vi "MicroblazeHostExample.vi"() -> ()   [LabVIEW 2015]
uses:
  <vilib>/userdefined/High Color/nirio_resource_hc.ctl
  <vilib>/FPGAPlugInAG/PXIe-6592R/niLvFpga_Open_PXIe-6592R.vi
  <vilib>/rvi/interface/common/dynamic/niFpgaDynamicAddResources.vi
  <vilib>/FPGAPlugInAG/Dynamic/niLvFpga_Reset_Dynamic.vi
  <vilib>/FPGAPlugInAG/Dynamic/niLvFpga_Download_Dynamic.vi
  <vilib>/FPGAPlugInAG/Dynamic/niLvFpga_Run_Dynamic.vi
  <vilib>/Utility/error.llb/Error Cluster From Error Code.vi
  <vilib>/rvi/errors/niLvFpgaAdjustHostInterfaceError.vi
  <vilib>/FPGAPlugInAG/Dynamic/niLvFpga_Close_Dynamic.vi
  <vilib>/rvi/interface/nirviOpenFPGA/nirviOpenFPGA.xnode
  FPGA Bitfiles/working/Microblaze.lvbitx
  <vilib>/rvi/interface/nirviMethod/nirviMethod.xnode
  <vilib>/rvi/interface/nirviReadWriteControl/nirviReadWriteControl.xnode
  <vilib>/rvi/interface/nirviCloseFPGA/nirviCloseFPGA.xnode
  <vilib>/rvi/interface/Simulation/niFpgaSimulationCallBeginRW.vi
  NiFpgaLv.dll
panel:
  in  "Flush Console":bool
  out "error out":errorcluster
  in  "FPGA Resource Name":T1="PXI1Slot6"
  out "UART Console":string="Goodbye cruel World\r\n"
  out "C":u32=12
  in  "B":u32=6
  in  "A":u32=2
  in  "C Code Executable to Download":path=path "C:/Users/8135cont24/Documents/CodeDistribution/LVFPGAHost/MicroBlazeELFFiles/helloworld1.elf"
  in  "Download C Code":bool
  in  "Stop":bool
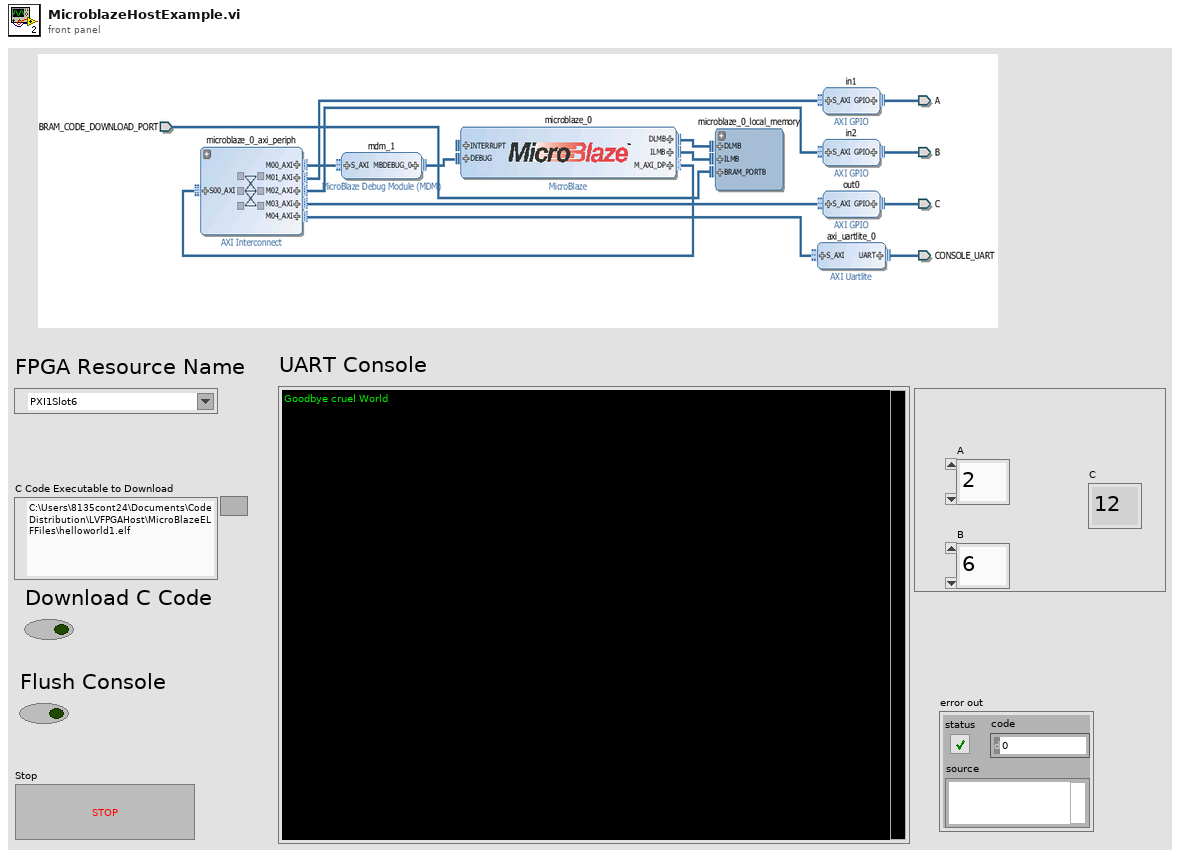
[diagram p1: front panel]
types:
  T1 = typedef "nirio_resource_hc.ctl" = tag
  T2 = cluster{"Baud (ticks)":u32, "CharacterSize":u8, "Parity":enum8{"None", "Even", "Odd"}, "Stop Bits":enum8{"1.0", "1.5", "2.0"}, "Spacing (ticks)":u32}
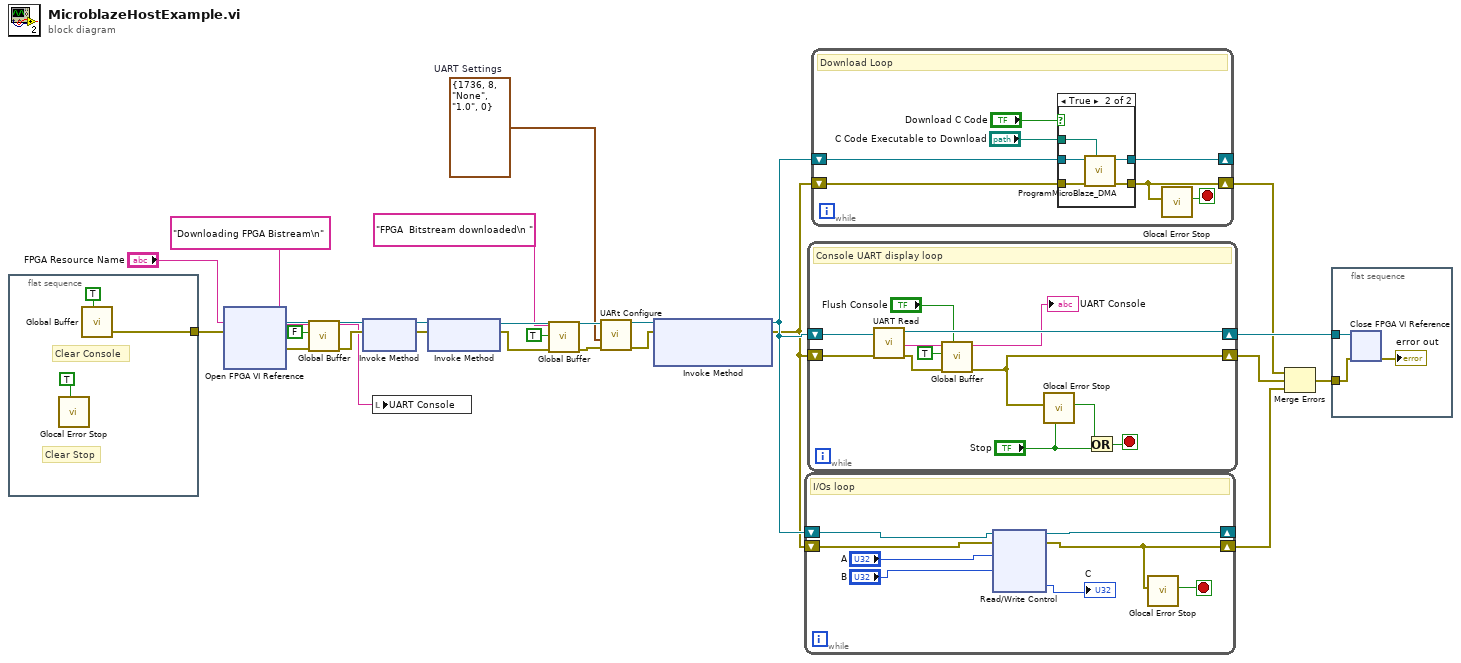
[diagram p0: block diagram]
diagram:
  w6 = T2 {"Baud (ticks)"=1736, "CharacterSize"=8, "Parity"=enum."None", "Stop Bits"=enum."1.0", "Spacing (ticks)"=0}  # UART Settings
  n1 = flat-sequence {
    tunnel: [w26] -> w14
    frame #0 {
      # "Clear Console"
      # "Clear Stop"
      n2 = call "Glocal Error Stop.vi"("Clear"=TRUE ("MainLoopStopped")) -> ()  [unwired: 10 in, 1 out]
      n3 = call "Global Buffer.vi"("Clear"=TRUE) -> ("Error Out"=w26:errorcluster)  [unwired: 9 in, 1 out]
    }
  }
  n4 = xnode "Open FPGA VI Reference"("error in"=w14, "resource name"="FPGA Resource Name") -> ("FPGA VI Reference Out"=w19:refnum<k20>, "error out"=w4:errorcluster)
  n5 = call "Global Buffer.vi"("Error In"=w4, "Append"=FALSE, "Input String"="Downloading FPGA Bistream\n" ("string")) -> ("Error Out"=w5:errorcluster, "Output String"=w1:string)  [unwired: 7 in]
  n6 = xnode "Invoke Method"("FPGA VI Reference In"=w19, "error in"=w5) -> ("FPGA VI Reference Out"=w21:refnum<k20>, "error out"=w20:errorcluster)
  n7 = local write "UART Console"(w1) -> ()
  n8 = xnode "Invoke Method"("FPGA VI Reference In"=w21, "error in"=w20) -> ("FPGA VI Reference Out"=w18:refnum<k20>, "error out"=w10:errorcluster)
  n9 = call "Global Buffer.vi"("Error In"=w10, "Append"=TRUE, "Input String"="FPGA  Bitstream downloaded\n " ("string")) -> ("Error Out"=w9:errorcluster)  [unwired: 7 in, 1 out]
  n10 = call "UARt Configure.vi"("Error In"=w9, "UART Settings"=w6, "FPGA Interface"=w18) -> ("Error Out"=w11:errorcluster, "FPGA Interface Out"=w12:refnum<k20>)  [unwired: 7 in]
  n11 = xnode "Invoke Method"("FPGA VI Reference In"=w12, "error in"=w11) -> ("FPGA VI Reference Out"=w24:refnum<k20>, "error out"=w15:errorcluster)  [unwired: 1 in]
  n12 = while {
    shift-right: [w33] -> w16
    shift-left: w15 -> [w34]
    shift-right: [w35] -> _
    shift-left: w24 -> [w36]
    stop <- w32 stop-if-true
    # "I/Os loop"
    n13 = xnode "Read/Write Control"("FPGA VI Reference In"=w36, "error in"=w34, "A"="A", "B"="B") -> ("FPGA VI Reference Out"=w35:refnum<k20>, "error out"=w33:errorcluster, "C"=→"C":u32)
    n14 = call "Glocal Error Stop.vi"("Error In"=w33) -> ("Output"=w32:bool)  [unwired: 10 in]
  }
  n15 = while {
    shift-right: [w48] -> w25
    shift-left: w24 -> [w44]
    shift-right: [w41] -> w22
    shift-left: w15 -> [w43]
    stop <- w46 stop-if-true
    # "Console UART display loop"
    n16 = call "UART Read.vi"("Error In"=w43, "FPGA Interface"=w44) -> ("Error Out"=w42:errorcluster, "UART Console"=w39:string, "FPGA Interface Out"=w48:refnum<k20>)  [unwired: 7 in]
    n17 = call "Global Buffer.vi"("Clear"="Flush Console", "Error In"=w42, "Append"=TRUE, "Input String"=w39) -> ("Error Out"=w41:errorcluster, "Output String"=→"UART Console":string)  [unwired: 6 in]
    n18 = call "Glocal Error Stop.vi"("Force Stop"="Stop", "Error In"=w41) -> ("Output"=w47:bool)  [unwired: 9 in]
    n19 = Or(x=w47, y="Stop") -> (x .or. y?=w46:bool)
  }
  n20 = while {
    shift-right: [w52] -> _
    shift-left: w24 -> [w54]
    shift-right: [w51] -> w13
    shift-left: w15 -> [w53]
    stop <- w50 stop-if-true
    # "Download Loop"
    n21 = case shown="True" "Download C Code" {
      tunnel: w54 -> [w56 w62]
      tunnel: [w57 w61] -> w51
      tunnel: w53 -> [w57 w59]
      tunnel: [w56 w60] -> w52
      tunnel: "C Code Executable to Download" -> [_ w58]
      frame False {
      }
      frame True {
        n22 = call "ProgramMicroBlaze_DMA.vi"("Elf File to Download"=w58, "error in (no error)"=w59, "FPGA Interface"=w62) -> ("error out"=w61:errorcluster, "FPGA Interface Out"=w60:refnum<k20>)  [unwired: 6 in, 1 out]
      }
    }
    n23 = call "Glocal Error Stop.vi"("Error In"=w51) -> ("Output"=w50:bool)  [unwired: 10 in]
  }
  n24 = Merge Errors(w13, w22, w16) -> (w23:errorcluster)
  n25 = flat-sequence {
    tunnel: w25 -> [w65]
    tunnel: w23 -> [w64]
    frame #0 {
      n26 = xnode "Close FPGA VI Reference"("FPGA VI Reference In"=w65, "error in"=w64) -> ("error out"=→"error out":errorcluster)
    }
  }
